vi "Cargo conditioning.vi"(10 "Cargo Out (Axis)":dbl, 11 "Cargo In (Axis)":dbl) -> (2 "Cargo Out (Hold)":bool, 3 "Cargo In (Hold)":bool)   [LabVIEW 2018, in "Joysticks.lvlib" / "Joysticks.lvclass"]
uses:
  Joysticks.lvclass
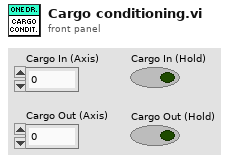
[diagram p1: front panel]
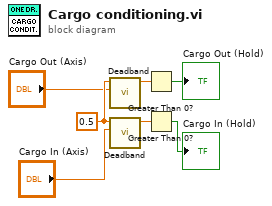
[diagram p0: block diagram]
diagram:
  w7 = 0.5 ("DeadBand")
  n1 = call "Deadband.vi"("joystick axis"="Cargo Out (Axis)", "DeadBand"=w7) -> ("Deadbanded output"=w4:dbl)  [unwired: 9 in]
  n2 = call "Deadband.vi"("joystick axis"="Cargo In (Axis)", "DeadBand"=w7) -> ("Deadbanded output"=w3:dbl)  [unwired: 9 in]
  n3 = Greater Than 0?(x=w4) -> (x > 0?=→"Cargo Out (Hold)":bool)
  n4 = Greater Than 0?(x=w3) -> (x > 0?=→"Cargo In (Hold)":bool)
